vi "profibus to tag bus.vi"(9 "Data in":u8[](array[numeric]), 10 "slave configuration":T2, 11 "data table in":T1) -> (3 "data table out":T1)   [LabVIEW 2013, in "Profibus Module runtime.lvclass"]
uses:
  Profibus Module runtime.lvclass
  profibus slave configuration.ctl
  profibus mapping configuration.ctl
  <vilib>/NI/Tag Bus/tag/Data Type.ctl
  dynamic profibus/full command.ctl
  dynamic profibus/profibus master action.ctl
  <vilib>/NI/Tag Bus/table/data table.ctl
  <vilib>/NI/Tag Bus/table/data polymorphs/write one/write Double.vi
  <vilib>/NI/Tag Bus/table/data polymorphs/write one/write Array of U8.vi
  <vilib>/NI/Tag Bus/table/data polymorphs/write one/write Array of U16.vi
  <vilib>/NI/Tag Bus/table/data polymorphs/write one/write Array of U32.vi
  <vilib>/NI/Tag Bus/table/data polymorphs/write one/write Single.vi
  <vilib>/NI/Tag Bus/table/data polymorphs/write one/write I32.vi
  <vilib>/NI/Tag Bus/table/data polymorphs/write one/write U32.vi
  <vilib>/NI/Tag Bus/table/data polymorphs/write one/write U16.vi
  <vilib>/NI/Tag Bus/table/data polymorphs/write one/write I16.vi
  <vilib>/NI/Tag Bus/table/data polymorphs/write one/write U8.vi
  <vilib>/NI/Tag Bus/table/data polymorphs/write one/write I8.vi
  <vilib>/NI/Tag Bus/table/data polymorphs/write one/write Boolean.vi
  <vilib>/NI/Tag Bus/table/data table.lvlib
  <vilib>/NI/Tag Bus/tag/tag descriptor.lvclass
  dynamic profibus/dynamic profibus.lvlib
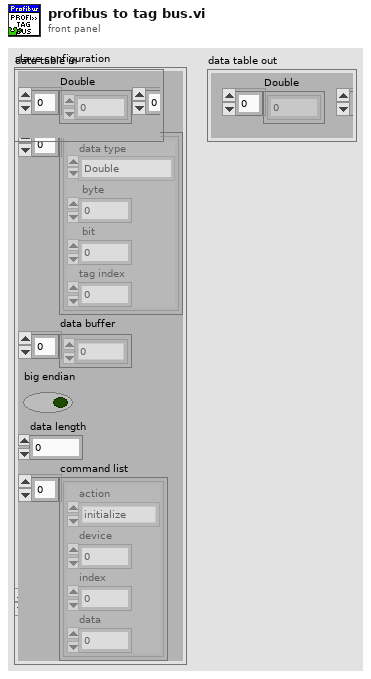
[diagram p1: front panel]
types:
  T1 = typedef "tag bus.lvlib/data table.lvlib/data table.ctl" = cluster{"Double":dbl[], "Single":sgl[], "I64":i64[], "I32":i32[], "I16":i16[], "I8":i8[], "U64":u64[], "U32":u32[], "U16":u16[], "U8":u8[], "Boolean":bool[], "String":string[], "Array of Double":cluster{"DBL Array":dbl[]}[], "Array of Single":cluster{"SGL Array":sgl[]}[], "Array of I64":cluster{"I64 Array":i64[]}[], "Array of I32":cluster{"I32 Array":i32[]}[], "Array of I16":cluster{"I16 Array":i16[]}[], "Array of I8":cluster{"I8 Array":i8[]}[], "Array of U64":cluster{"U64 Array":u64[]}[], "Array of U32":cluster{"U32 Array":u32[]}[], "Array of U16":cluster{"U16 Array":u16[]}[], "Array of U8":cluster{"U8 Array":u8[]}[], "Array of Boolean":cluster{"Boolean Array":bool[]}[], "Array of String":cluster{"String Array":string[]}[]}
  T2 = typedef "Profibus Module runtime.lvclass/profibus slave configuration.ctl" = cluster{"slave index":i8, "data items":T3[], "data buffer":u8[], "big endian":bool, "data length":i32, "command list":T5[]}
  T3 = typedef "Profibus Module runtime.lvclass/profibus mapping configuration.ctl" = cluster{"data type":T4, " byte":i32, " bit":i32, "tag index":i32}
  T4 = typedef "tag bus.lvlib/tag descriptor.lvclass/Data Type.ctl" = enum16{"Double", "Single", "I64", "I32", "I16", "I8", "U64", "U32", "U16", "U8", "Boolean", "String", "Array of Double", "Array of Single", "Array of I64", "Array of I32", "Array of I16", "Array of I8", "Array of U64", "Array of U32", "Array of U16", "Array of U8", "Array of Boolean", "Array of String"}
  T5 = typedef "dynamic profibus.lvlib/full command.ctl" = cluster{"action":T6, "device":u8, "index":u8, "data":u8}
  T6 = typedef "dynamic profibus.lvlib/profibus master action.ctl" = enum8{"initialize", "uninitialize", "stop", "get input", "get input size", "set output", "get output size", "get diagnostic", "transfer data", "transfer diagnostics"}
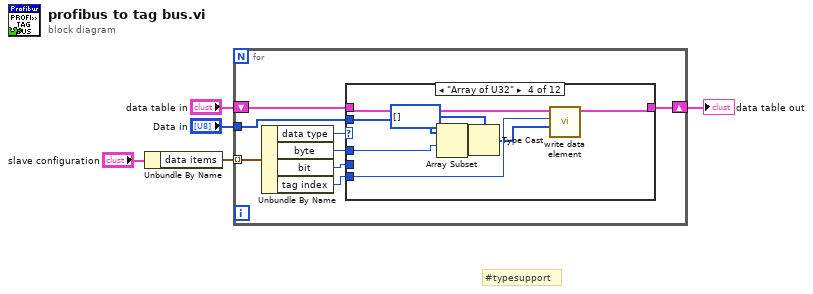
[diagram p0: block diagram]
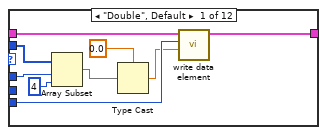
[diagram p2: hidden frame]
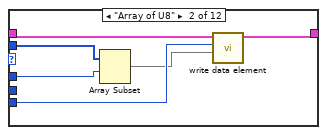
[diagram p3: hidden frame]
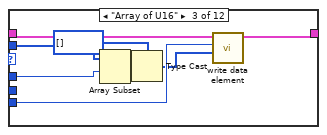
[diagram p4: hidden frame]
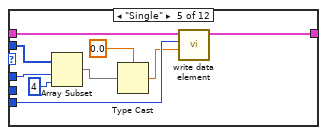
[diagram p5: hidden frame]
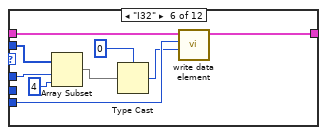
[diagram p6: hidden frame]
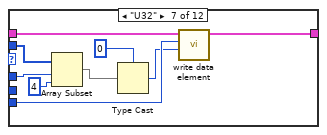
[diagram p7: hidden frame]
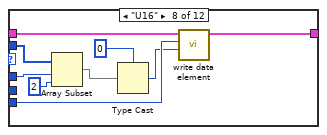
[diagram p8: hidden frame]
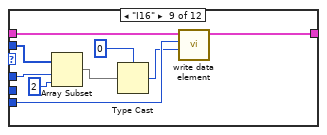
[diagram p9: hidden frame]
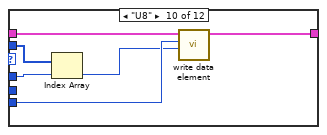
[diagram p10: hidden frame]
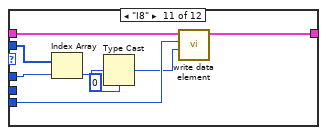
[diagram p11: hidden frame]
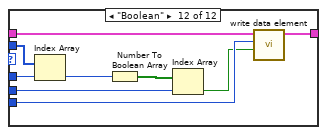
[diagram p12: hidden frame]
diagram:
  # "#typesupport"
  n1 = Unbundle By Name("slave configuration") -> ("data items"=w4:T3[])
  n2 = for {
    tunnel: w4 -> [w13] mode=indexing
    tunnel: "Data in" -> [w10]
    shift-right: [w7] -> w2
    shift-left: "data table in" -> [w6]
    n3 = Unbundle By Name(w13) -> ("data type"=w12:T4, "byte"=w11:i32, "bit"=w9:i32, "tag index"=w8:i32)
    n4 = case shown="\"Array of U32\"" w12 {
      tunnel: w10 -> [w22 w26 w34 w42 w53 w62 w71 w80 w89 w95 w103 w112]
      tunnel: w11 -> [w21 w25 w33 w41 w52 w61 w70 w79 w88 w94 w102 w111]
      tunnel: w9 -> [_ _ _ _ _ _ _ _ _ _ _ w108]
      tunnel: w8 -> [w17 w24 w32 w40 w48 w57 w66 w75 w84 w93 w101 w105]
      tunnel: [w15 w27 w35 w43 w46 w55 w64 w73 w82 w92 w100 w107] -> w7
      tunnel: w6 -> [w14 w28 w36 w44 w45 w54 w63 w72 w81 w91 w99 w106]
      frame "Double", Default {
        n5 = Array Subset(array=w22, index=w21, length=4) -> (w19:u8[])
        n6 = Type Cast(type=sgl 0.0, x=w19) -> (*(type *) &x=w16:sgl)
        n7 = call-poly <vilib>:"write data element.vi"("value"=w16, "index"=w17, "data table in"=w14) -> ("data table out"=w15:T1)  [unwired: 8 in]
      }
      frame "Array of U8" {
        n8 = Array Subset(array=w26, index=w25) -> (w23:u8[])  [unwired: 1 in]
        n9 = call-poly <vilib>:"write data element.vi"("value"=w23, "index"=w24, "data table in"=w28) -> ("data table out"=w27:T1)  [unwired: 8 in]
      }
      frame "Array of U16" {
        n10 = Array Subset(array=w34, index=w33) -> (w31:u8[])  [unwired: 1 in]
        n11 = Type Cast(type=u16[] [] ("value"), x=w31) -> (*(type *) &x=w29:u16[])
        n12 = call-poly <vilib>:"write data element.vi"("value"=w29, "index"=w32, "data table in"=w36) -> ("data table out"=w35:T1)  [unwired: 8 in]
      }
      frame "Array of U32" {
        n13 = Array Subset(array=w42, index=w41) -> (w39:u8[])  [unwired: 1 in]
        n14 = Type Cast(type=u32[] [] ("value"), x=w39) -> (*(type *) &x=w37:u32[])
        n15 = call-poly <vilib>:"write data element.vi"("value"=w37, "index"=w40, "data table in"=w44) -> ("data table out"=w43:T1)  [unwired: 8 in]
      }
      frame "Single" {
        n16 = Array Subset(array=w53, index=w52, length=4) -> (w50:u8[])
        n17 = Type Cast(type=sgl 0.0, x=w50) -> (*(type *) &x=w47:sgl)
        n18 = call-poly <vilib>:"write data element.vi"("value"=w47, "index"=w48, "data table in"=w45) -> ("data table out"=w46:T1)  [unwired: 8 in]
      }
      frame "I32" {
        n19 = Array Subset(array=w62, index=w61, length=4) -> (w59:u8[])
        n20 = Type Cast(type=0, x=w59) -> (*(type *) &x=w56:i32)
        n21 = call-poly <vilib>:"write data element.vi"("value"=w56, "index"=w57, "data table in"=w54) -> ("data table out"=w55:T1)  [unwired: 8 in]
      }
      frame "U32" {
        n22 = Array Subset(array=w71, index=w70, length=4) -> (w68:u8[])
        n23 = Type Cast(type=u32 0, x=w68) -> (*(type *) &x=w65:u32)
        n24 = call-poly <vilib>:"write data element.vi"("value"=w65, "index"=w66, "data table in"=w63) -> ("data table out"=w64:T1)  [unwired: 8 in]
      }
      frame "U16" {
        n25 = Array Subset(array=w80, index=w79, length=2) -> (w77:u8[])
        n26 = Type Cast(type=u16 0, x=w77) -> (*(type *) &x=w74:u16)
        n27 = call-poly <vilib>:"write data element.vi"("value"=w74, "index"=w75, "data table in"=w72) -> ("data table out"=w73:T1)  [unwired: 8 in]
      }
      frame "I16" {
        n28 = Array Subset(array=w89, index=w88, length=2) -> (w86:u8[])
        n29 = Type Cast(type=i16 0, x=w86) -> (*(type *) &x=w83:i16)
        n30 = call-poly <vilib>:"write data element.vi"("value"=w83, "index"=w84, "data table in"=w81) -> ("data table out"=w82:T1)  [unwired: 8 in]
      }
      frame "U8" {
        n31 = Index Array(array=w95, index=w94) -> (element=w90:u8)
        n32 = call-poly <vilib>:"write data element.vi"("value"=w90, "index"=w93, "data table in"=w91) -> ("data table out"=w92:T1)  [unwired: 8 in]
      }
      frame "I8" {
        n33 = Index Array(array=w103, index=w102) -> (element=w98:u8)
        n34 = Type Cast(type=i8 0, x=w98) -> (*(type *) &x=w97:i8)
        n35 = call-poly <vilib>:"write data element.vi"("value"=w97, "index"=w101, "data table in"=w99) -> ("data table out"=w100:T1)  [unwired: 8 in]
      }
      frame "Boolean" {
        n36 = Index Array(array=w112, index=w111) -> (element=w110:u8)
        n37 = Number To Boolean Array(number=w110) -> (Boolean array=w109:bool[])
        n38 = Index Array(array=w109, index=w108) -> (element=w104:bool)
        n39 = call-poly <vilib>:"write data element.vi"("value"=w104, "index"=w105, "data table in"=w106) -> ("data table out"=w107:T1)  [unwired: 8 in]
      }
    }
  }
  "data table out" <- w2
